vi "ZigZagRole.vi"(8 "error in (no error)":errorcluster, 9 "Game in":refnum<class "Game.lvclass">, 10 "Robot in":refnum<class "Robot.lvclass">, 11 "ZigZagRole in":refnum<class "ZigZagRole.lvclass">) -> (0 "error out":errorcluster, 1 "Game out":refnum<class "Game.lvclass">, 2 "Robot out":refnum<class "Robot.lvclass">, 3 "ZigZagRole out":refnum<class "ZigZagRole.lvclass">)   [LabVIEW 2018, in "ZigZagRole.lvclass"]
uses:
  ZigZagRole.lvclass
  C:/Users/nicolas.oliveira/roboime/SSL_AI/Role_class/Role.lvclass
  Robot_class/Robot.lvclass
  Game_class/Game.lvclass
  Role_class/Role.lvclass/Role.ctl
  Tacticbook_class/Tacticbook.lvclass/Tacticbook.ctl
  Tacticbook_class/Read ZigZagTactic.vi
  ZigZagTactic_class/Read States.vi
  Tacticbook_class/Write ZigZagTactic.vi
  Role_class/Read Tacticbook.vi
  Role_class/Read tactic_index.vi
  Role_class/Write Tacticbook.vi
  Role_class/Write tactic_index.vi
  Tacticbook_class/Tacticbook.lvclass
  ZigZagTactic_class/ZigZagTactic.lvclass
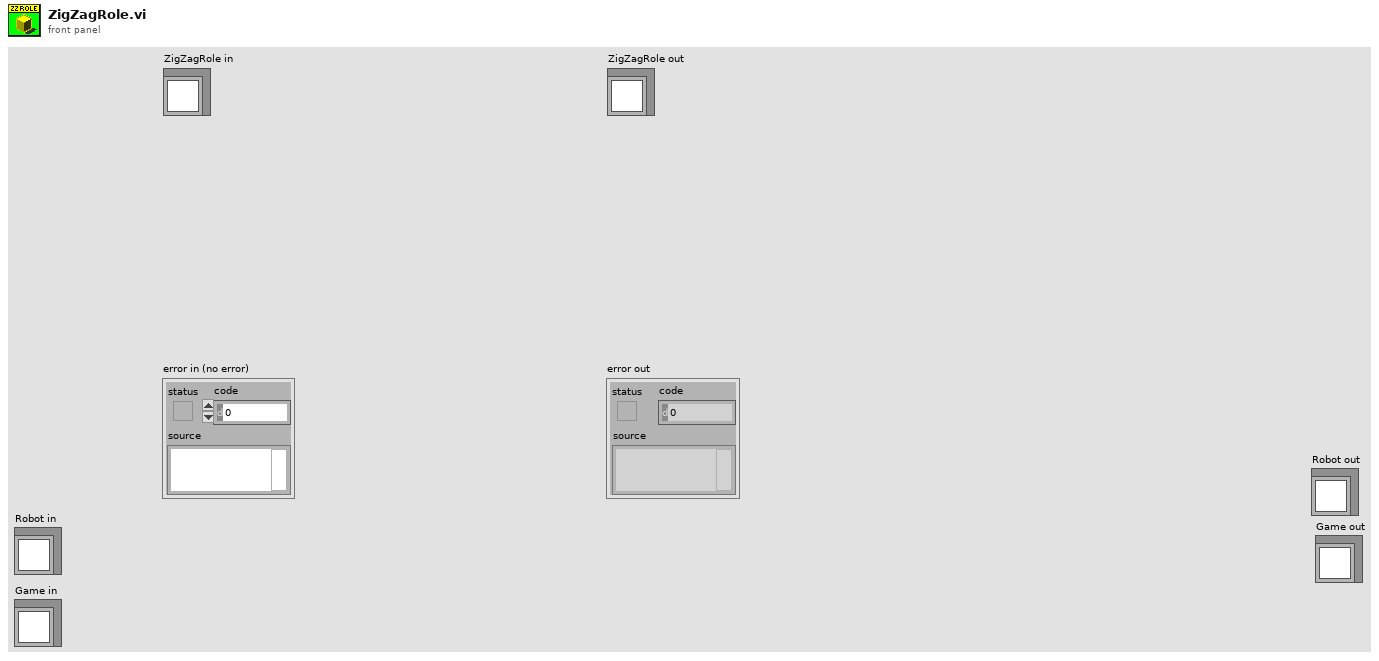
[diagram p1: front panel]
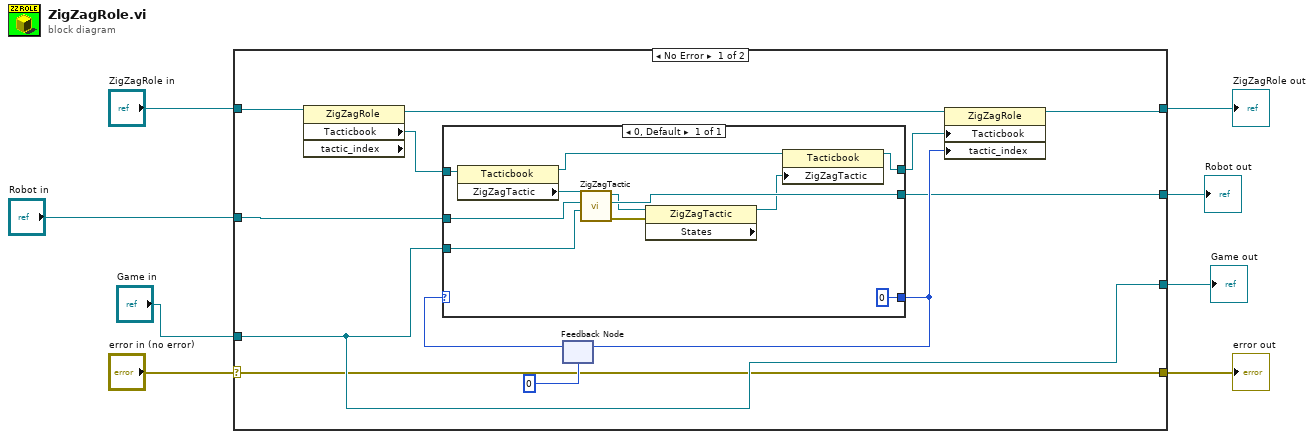
[diagram p0: block diagram]
diagram:
  n1 = case shown="No Error" "error in (no error)" {
    selector: "error in (no error)" -> [w9 w35]
    tunnel: [w9 w35] -> w7
    tunnel: [w13 w34] -> w5
    tunnel: "ZigZagRole in" -> [w14 w34]
    tunnel: "Robot in" -> [w12 w33]
    tunnel: "Game in" -> [w10 w32]
    tunnel: [w11 w33] -> w3
    tunnel: [w10 w32] -> w2
    frame No Error {
      n2 = property class="ZigZagRole" props=["Tacticbook", "tactic_index"](reference=w14) -> (reference out=w20:refnum<class "ZigZagRole.lvclass">, "Tacticbook"=w17:refnum<class "Tacticbook.lvclass">)  [unwired: 1 in, 2 out]
      n3 = feedback #1(0) -> (w18:i32)
      n4 = case shown="0, Default" w18 {
        tunnel: [0] -> w16
        tunnel: w17 -> [w31]
        tunnel: w12 -> [w22]
        tunnel: [w30] -> w11
        tunnel: [w26] -> w15
        tunnel: w10 -> [w21]
        frame 0, Default {
          n5 = property class="Tacticbook"(reference=w31) -> (reference out=w28:refnum<class "Tacticbook.lvclass">, "ZigZagTactic"=w25:refnum<class "ZigZagTactic.lvclass">)  [unwired: 1 in, 1 out]
          n6 = call-dynamic "ZigZagTactic.vi"("Game in"=w21, "Robot"=w22, "ZigZagTactic in"=w25) -> ("error out"=w29:errorcluster, "Robot out"=w30:refnum<class "Robot.lvclass">, "ZigZagTactic out"=w24:refnum<class "ZigZagTactic.lvclass">)  [unwired: 6 in]
          n7 = property class="ZigZagTactic" props=["States"](reference=w24, error in=w29) -> (reference out=w27:refnum<class "ZigZagTactic.lvclass">)  [unwired: 2 out]
          n8 = property class="Tacticbook"(reference=w28, "ZigZagTactic"=w27) -> (reference out=w26:refnum<class "Tacticbook.lvclass">)  [unwired: 1 in, 1 out]
        }
      }
      n9 = feedback-in #1(w16) -> ()
      n10 = property class="ZigZagRole"(reference=w20, "Tacticbook"=w15, "tactic_index"=w16) -> (reference out=w13:refnum<class "ZigZagRole.lvclass">)  [unwired: 1 in, 1 out]
    }
    frame Error {
    }
  }
  "error out" <- w7
  "ZigZagRole out" <- w5
  "Robot out" <- w3
  "Game out" <- w2
